vi "Video File Open.vi"(8 "error in (no error)":errorcluster, 10 "Path (\"\")":path, 11 "Video Processor in":refnum<class "Video Processor.lvclass">) -> (0 "error out":errorcluster, 3 "Video Processor out":refnum<class "Video Processor.lvclass">)   [LabVIEW 2018, in "Video Processor.lvclass"]
uses:
  Video Processor.lvclass
  <vilib>/vision/Avi.llb/IMAQ AVI2 Codec Path.ctl
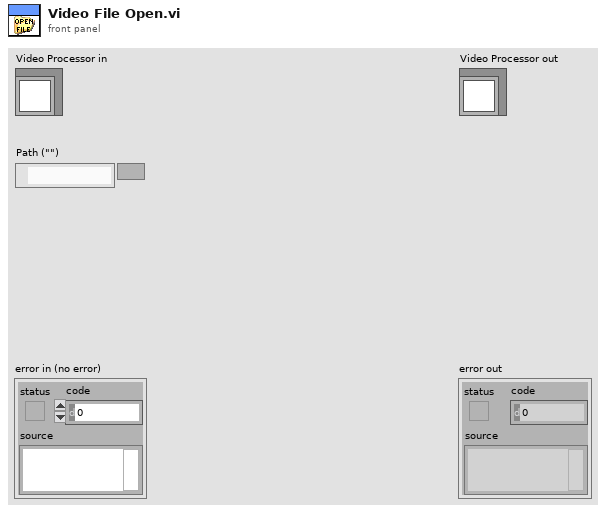
[diagram p1: front panel]
types:
  T1 = typedef "Image Type" = u32
  T2 = typedef "IMAQ AVI2 Codec Path.ctl" = u32
  T3 = typedef "IMAQ AVI2 Refnum.ctl" = refnum<k20>
  T4 = cluster{"Width":u32, "Height":u32, "Frames Per Second":u32, "Codec":string, "Has Data":bool}
  T5 = typedef "IMAQ Image.ctl" = refnum<image>
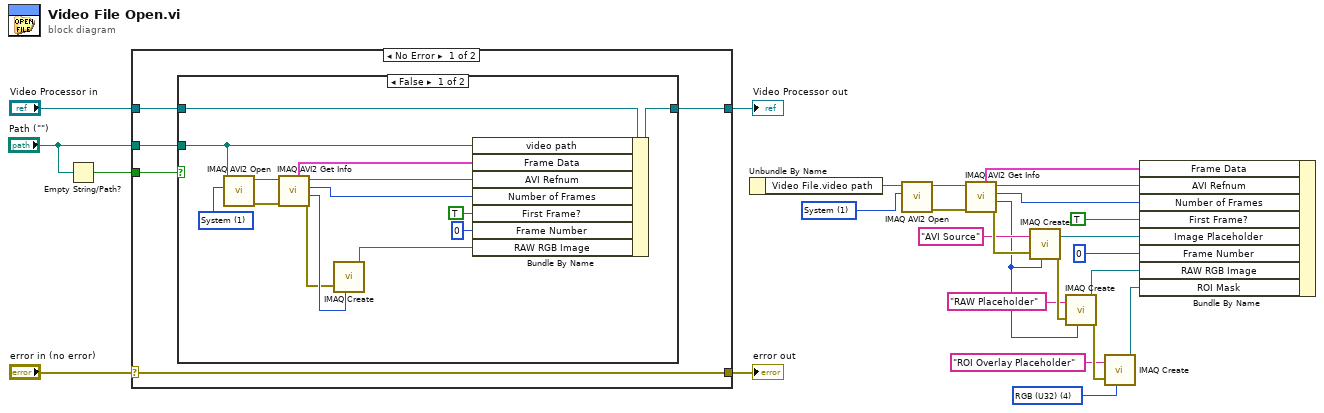
[diagram p0: block diagram]
diagram:
  w2 = T1 4 items=["Grayscale (U8)", "Grayscale (I16)", "Grayscale (SGL)", "Complex (CSG)", "RGB (U32)", "HSL (U32)", "RGB (U64)", "Grayscale (U16)"] ("Image Type")
  w10 = T2 1 items=["Default", "System", "Built in Vision"] ("Codec Source")
  n1 = Empty String/Path?(string/path="Path (\"\")") -> (empty?=w24:bool)
  n2 = case shown="No Error" "error in (no error)" {
    selector: "error in (no error)" -> [w34 w51]
    tunnel: [w34 w51] -> w28
    tunnel: [w30 w50] -> w26
    tunnel: "Video Processor in" -> [w31 w50]
    tunnel: "Path (\"\")" -> [w32 _]
    tunnel: w24 -> [w33 _]
    frame No Error {
      n3 = case shown="False" w33 {
        tunnel: w32 -> [w45 _]
        tunnel: w31 -> [w48 w49]
        tunnel: [w47 w49] -> w30
        frame False {
          w46 = T2 1 items=["Default", "System", "Built in Vision"] ("Codec Source")
          n4 = call "IMAQ AVI2 Open"("Codec Source"=w46, "AVI File Path"=w45) -> ("error out"=w43:errorcluster, "AVI Refnum"=w44:T3)  [unwired: 1 in, 7 out]
          n5 = call "IMAQ AVI2 Get Info"("error in (no error)"=w43, "AVI Refnum"=w44) -> ("error out"=w35:errorcluster, "Image Type"=w36:T1, "Number of Frames"=w40:u32, "AVI Refnum (duplicate)"=w41:T3, "Frame Data"=w42:T4)  [unwired: 5 out]
          n6 = call "IMAQ Create"("Image Type"=w36, "error in (no error)"=w35) -> ("New Image"=w37:T5)  [unwired: 2 in, 2 out]
          n7 = Bundle By Name(cluster=w48, "video path"=w45, "Frame Data"=w42, "AVI Refnum"=w41, "Number of Frames"=w40, "First Frame?"=TRUE ("Video File.First Frame?"), "Frame Number"=u32 0 ("Video File.Frame Number"), "RAW RGB Image"=w37) -> (w47:refnum<class "Video Processor.lvclass">)
        }
        frame True {
        }
      }
    }
    frame Error {
    }
  }
  "error out" <- w28
  "Video Processor out" <- w26
  n8 = Unbundle By Name() -> ("Video File.video path"=w22:path)  [unwired: 1 in]
  n9 = call "IMAQ AVI2 Open"("Codec Source"=w10, "AVI File Path"=w22) -> ("error out"=w19:errorcluster, "AVI Refnum"=w18:T3, "error in (no error)"=w23:errorcluster)  [unwired: 7 out]
  n10 = call "IMAQ AVI2 Get Info"("error in (no error)"=w19, "AVI Refnum"=w18) -> ("error out"=w14:errorcluster, "Image Type"=w7:T1, "Number of Frames"=w16:u32, "AVI Refnum (duplicate)"=w17:T3, "Frame Data"=w9:T4)  [unwired: 5 out]
  n11 = call "IMAQ Create"("Image Name"="AVI Source", "Image Type"=w7, "error in (no error)"=w14) -> ("New Image"=w12:T5, "error out"=w8:errorcluster)  [unwired: 1 in, 1 out]
  n12 = call "IMAQ Create"("Image Name"="RAW Placeholder", "Image Type"=w7, "error in (no error)"=w8) -> ("New Image"=w5:T5, "error out"=w4:errorcluster)  [unwired: 1 in, 1 out]
  n13 = call "IMAQ Create"("Image Name"="ROI Overlay Placeholder", "Image Type"=w2, "error in (no error)"=w4) -> ("New Image"=w1:T5)  [unwired: 1 in, 2 out]
  n14 = Bundle By Name("Frame Data"=w9, "AVI Refnum"=w17, "Number of Frames"=w16, "First Frame?"=TRUE, "Image Placeholder"=w12, "Frame Number"=u32 0, "RAW RGB Image"=w5, "ROI Mask"=w1) -> (w20:cluster{}, w21:cluster{})
